vi "ConfigureChannelsForStartupMeas.vi"(8 "error in (no error)":errorcluster, 9 "metric cache":variant, 10 "DataGroup":T1, 11 "device":T9) -> (0 "error out":errorcluster, 3 "valid channels for startup measurement":T6[](array[typedef]))   [LabVIEW 2017, in "McsaStartupAnalysis.lvlib"]
uses:
  <vilib>/addons/InsightCM/Devices/Shared/Mcsa/McsaStartupAnalysis/McsaStartupAnalysis.lvlib
  <vilib>/addons/InsightCM/MessageBus/Base/controls/R2_DeviceModel.ctl
  <vilib>/addons/InsightCM/MessageBus/Base/controls/R2_Device.ctl
  <vilib>/addons/InsightCM/MessageBus/Base/controls/KeyValuePair.ctl
  <vilib>/addons/InsightCM/MessageBus/Base/controls/DeviceState.ctl
  <vilib>/addons/InsightCM/MessageBus/Base/controls/R2_DataGroup.ctl
  <vilib>/addons/InsightCM/MessageBus/Base/controls/OperatingState.ctl
  <vilib>/addons/InsightCM/MessageBus/Base/controls/Trigger.ctl
  <vilib>/addons/InsightCM/MessageBus/Base/controls/Condition.ctl
  <vilib>/addons/InsightCM/MessageBus/Base/controls/BurstModeTrigger.ctl
  <vilib>/addons/InsightCM/MessageBus/Base/controls/R2_Channel.ctl
  <vilib>/addons/InsightCM/MessageBus/Base/controls/Metric.ctl
  <vilib>/addons/InsightCM/MessageBus/Base/controls/Tag.ctl
  <vilib>/addons/InsightCM/Devices/Shared/Mcsa/McsaStartupAnalysis/controls/ChannelForStartup.ctl
  <vilib>/addons/InsightCM/Devices/Shared/Mcsa/McsaStartupAnalysis/controls/StartupFeature.ctl
  <vilib>/addons/InsightCM/Devices/Shared/Mcsa/McsaStartupAnalysis/controls/MotorInfo.ctl
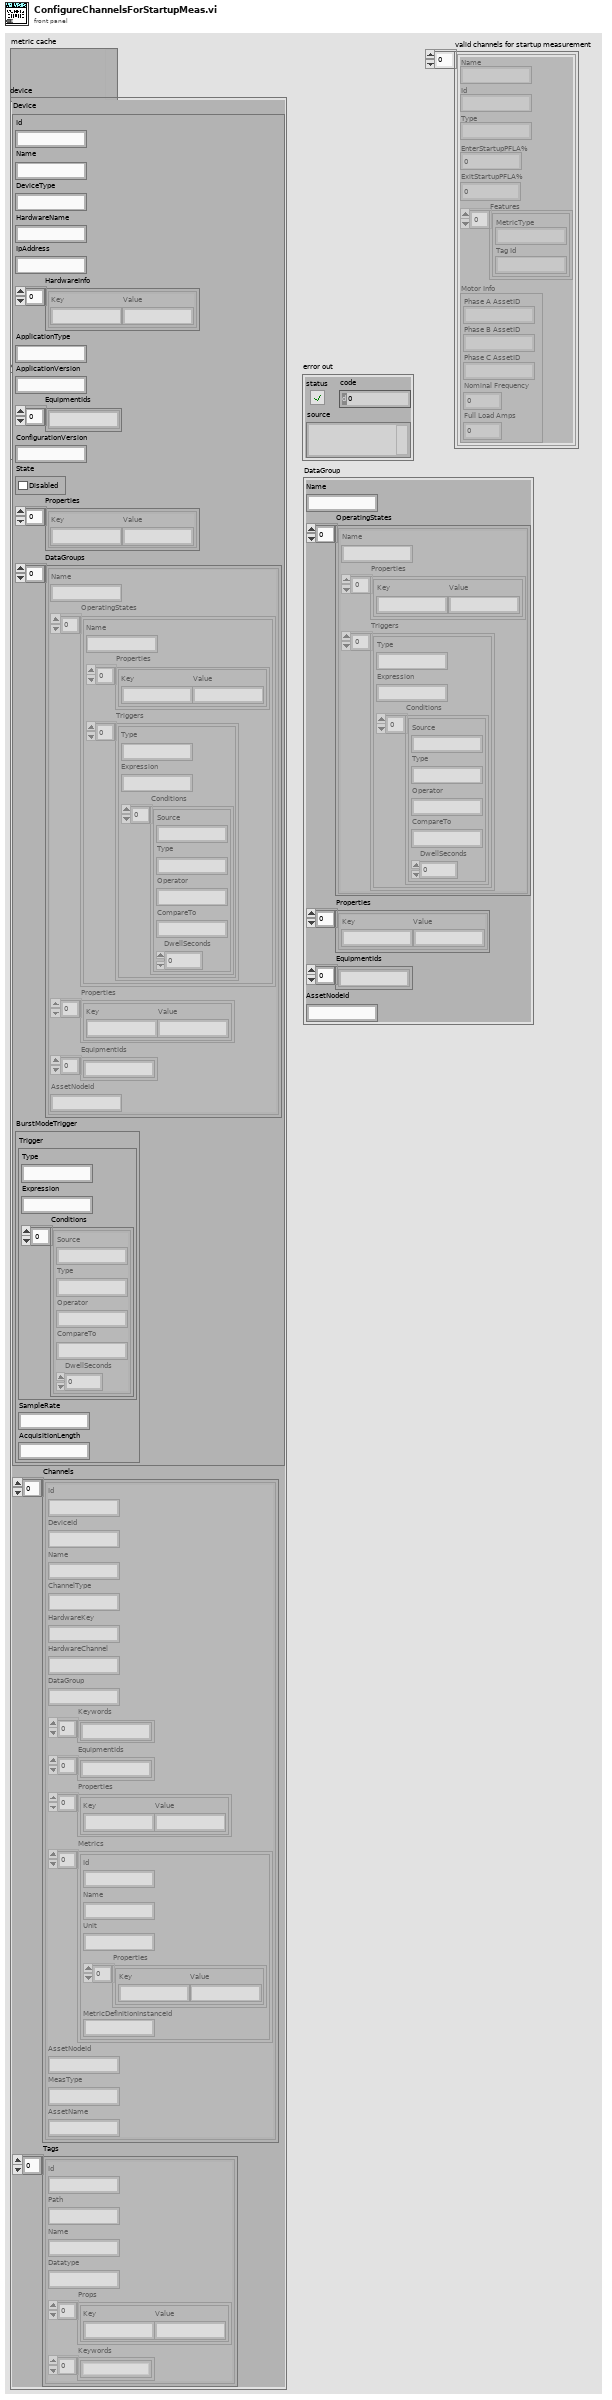
[diagram p1: front panel]
types:
  T1 = typedef "R2_DataGroup.ctl" = cluster{"Name":string, "OperatingStates":T2[], "Properties":T3[], "EquipmentIds":string[], "AssetNodeId":string}
  T2 = typedef "OperatingState.ctl" = cluster{"Name":string, "Properties":T3[], "Triggers":T4[]}
  T3 = typedef "KeyValuePair.ctl" = cluster{"Key":string, "Value":string}
  T4 = typedef "Trigger.ctl" = cluster{"Type":string, "Expression":string, "Conditions":T5[]}
  T5 = typedef "Condition.ctl" = cluster{"Source":string, "Type":string, "Operator":string, "CompareTo":string, "DwellSeconds":dbl}
  T6 = typedef "McsaStartupAnalysis.lvlib/ChannelForStartup.ctl" = cluster{"Name":string, "Id":string, "Type":string, "EnterStartupPFLA%":dbl, "ExitStartupPFLA%":dbl, "Features":T7[], "Motor Info":T8}
  T7 = typedef "McsaStartupAnalysis.lvlib/StartupFeature.ctl" = cluster{"MetricType":string, "Tag Id":string}
  T8 = typedef "McsaStartupAnalysis.lvlib/MotorInfo.ctl" = cluster{"Phase A AssetID":string, "Phase B AssetID":string, "Phase C AssetID":string, "Nominal Frequency":dbl, "Full Load Amps":dbl}
  T9 = typedef "R2_DeviceModel.ctl" = cluster{"Device":T10, "Channels":T13[], "Tags":T15[]}
  T10 = typedef "R2_Device.ctl" = cluster{"Id":string, "Name":string, "DeviceType":string, "HardwareName":string, "IpAddress":string, "HardwareInfo":T3[], "ApplicationType":string, "ApplicationVersion":string, "EquipmentIds":string[], "ConfigurationVersion":string, "State":T11, "Properties":T3[], "DataGroups":T1[], "BurstModeTrigger":T12}
  T11 = typedef "DeviceState.ctl" = cluster{"Disabled":bool}
  T12 = typedef "BurstModeTrigger.ctl" = cluster{"Trigger":T4, "SampleRate":string, "AcquisitionLength":string}
  T13 = typedef "R2_Channel.ctl" = cluster{"Id":string, "DeviceId":string, "Name":string, "ChannelType":string, "HardwareKey":string, "HardwareChannel":string, "DataGroup":string, "Keywords":string[], "EquipmentIds":string[], "Properties":T3[], "Metrics":T14[], "AssetNodeId":string, "MeasType":string, "AssetName":string}
  T14 = typedef "Metric.ctl" = cluster{"Id":string, "Name":string, "Unit":string, "Properties":T3[], "MetricDefinitionInstanceId":string}
  T15 = typedef "Tag.ctl" = cluster{"Id":string, "Path":string, "Name":string, "Datatype":string, "Props":T3[], "Keywords":string[]}
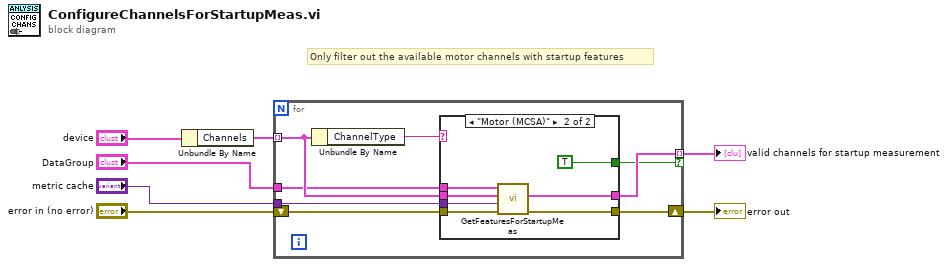
[diagram p0: block diagram]
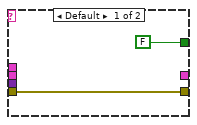
[diagram p2: hidden frame]
diagram:
  # "Only filter out the available motor channels with startup features"
  n1 = Unbundle By Name("device") -> ("Channels"=w4:T13[])
  n2 = for {
    tunnel: "metric cache" -> [w14]
    tunnel: w4 -> [w13] mode=indexing
    shift-right: [w11] -> w5
    shift-left: "error in (no error)" -> [w15]
    tunnel: [w10] -> w3 mode=indexing if=w9
    tunnel: "DataGroup" -> [w8]
    n3 = Unbundle By Name(w13) -> ("ChannelType"=w12:string)
    n4 = case shown="\"Motor (MCSA)\"" w12 {
      tunnel: w15 -> [w17 w24]
      tunnel: w14 -> [_ w23]
      tunnel: w13 -> [_ w19]
      tunnel: [_ w22] -> w10
      tunnel: [w17 w21] -> w11
      tunnel: [FALSE TRUE] -> w9
      tunnel: w8 -> [_ w18]
      frame Default {
      }
      frame "Motor (MCSA)" {
        n5 = call <vilib>:"GetFeaturesForStartupMeas.vi"("error in (no error)"=w24, "Metric Cache"=w23, "ChannelModel"=w19, "DataGroup"=w18) -> ("error out"=w21:errorcluster, "Channels for Startup"=w22:T6)  [unwired: 6 in]
      }
    }
  }
  "error out" <- w5
  "valid channels for startup measurement" <- w3
